vi "Batch Configure FP Window Size.vi"() -> ()   [LabVIEW 2025]
doc: "Instrument Driver Compliance Tool\n\nDescription:\nThe <b>Instrument Driver Compliance Tool</b> provides automated support for adjusting VI properties to meet the guidelines specified by NI in the Instrument Driver Development Tools and Resources. It ensures consistency across all driver VIs and reduces manual configuration effort.\n\nKey Rules Enforced:\n\n<b>Protection</b>: Unlocked — Users must have access to the source code for customization and extension.\n\n<b>Window Appearance</b>: Default — Guarantees consistent appearance with standard LabVIEW VIs.\n\n<b>Execution</b>:\n\nAllow Debugging: Enabled — Facilitates troubleshooting of cables, addresses, and configuration.\n\nReentrant Execution: Disabled — Avoids unnecessary memory overhead and simplifies debugging.\n\nPreferred Execution System: Same as Caller — Ensures flexibility according to application needs.\n\nAutomatic Error Handling: Disabled — Error management should be handled explicitly via error clusters.\n\nRun when Opened: Disabled — Execution should remain under user control.\n\nSuspend when Called: Disabled — Instrument Driver VIs must not suspend when invoked.\n\nUsage:\nRun this tool on VIs within an instrument driver project to validate or apply the recommended property settings automatically.\n\nBenefits:\n\nGuarantees NI-compliant driver development.\n\nSaves time by standardizing VI property settings.\n\nImproves maintainability and debugging capabilities."
uses:
  <vilib>/Utility/miscctls.llb/LVPointTypeDef.ctl
panel:
  in  "Front Panel Window:Minimum Size":T1={"Horizontal"=457, "Vertical"=288}
  in  "Folder VIs Path":path
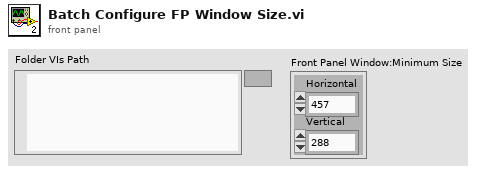
[diagram p1: front panel]
types:
  T1 = typedef "LVPointTypeDef.ctl" = cluster{"Horizontal":i16, "Vertical":i16}
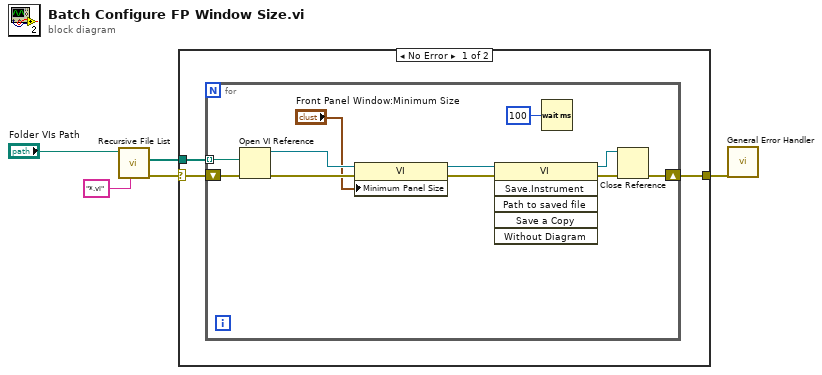
[diagram p0: block diagram]
diagram:
  n1 = call <vilib>:"Recursive File List.vi"("pattern"="*.vi", "Folder Path"="Folder VIs Path") -> ("error out"=w1:errorcluster, "All Files in Dir"=w4:path[])  [unwired: 5 in, 3 out]
  n2 = case shown="No Error" w1 {
    selector: w1 -> [w6 w20]
    tunnel: w4 -> [w8 _]
    tunnel: [w7 w20] -> w3
    frame No Error {
      n3 = for {
        tunnel: w8 -> [w19] mode=indexing
        shift-right: [w17] -> w7
        shift-left: w6 -> [w18]
        n4 = Open VI Reference(vi path=w19, error in (no error)=w18) -> (vi reference=w11:refnum<vi>, error out=w12:errorcluster)  [unwired: 4 in]
        n5 = property class="VI"(reference=w11, error in=w12, "Minimum Panel Size"="Front Panel Window:Minimum Size") -> (reference out=w14:refnum<vi>, error out=w10:errorcluster)
        n6 = invoke class="VI" method="Save.Instrument"(reference=w14, error in=w10) -> (reference out=w15:refnum<vi>, error out=w16:errorcluster)  [unwired: 4 in, 4 out]
        n7 = Wait (ms)(milliseconds to wait=u32 100) -> ()  [unwired: 1 out]
        n8 = Close Reference(reference=w15, error in (no error)=w16) -> (error out=w17:errorcluster)
      }
    }
    frame Error {
    }
  }
  n9 = call <vilib>:"General Error Handler.vi"("error in (no error)"=w3) -> ()  [unwired: 10 in, 5 out]
